vi "Read_fw_info.vi"(8 "error in (no error)":errorcluster, 11 "VISA Refnum in":refnum<visa-resource-name>) -> (0 "error out":errorcluster, 1 "Firmware Version":string, 2 "Hardware":string, 3 "VISA Refnum out":refnum<visa-resource-name>, 5 "Project":string)   [LabVIEW 2019]
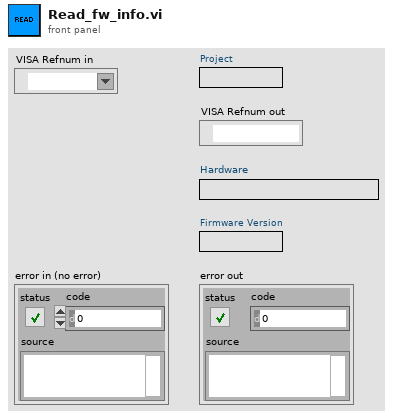
[diagram p1: front panel]
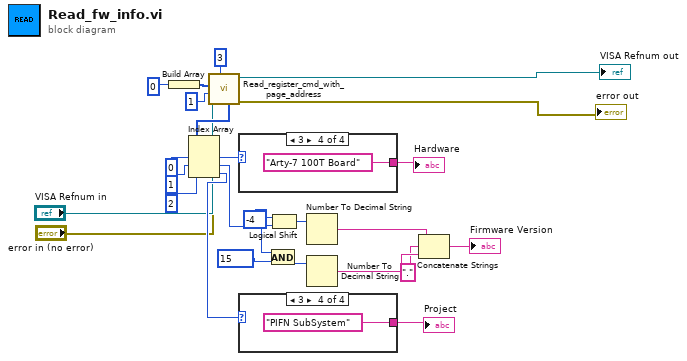
[diagram p0: block diagram]
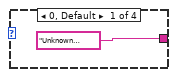
[diagram p2: hidden frame]
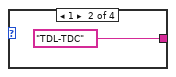
[diagram p3: hidden frame]
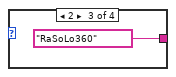
[diagram p4: hidden frame]
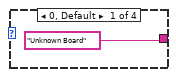
[diagram p5: hidden frame]
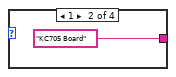
[diagram p6: hidden frame]
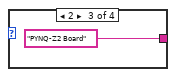
[diagram p7: hidden frame]
diagram:
  n1 = Build Array(u8 0) -> (w1:u8[])
  n2 = call "Read_register_cmd_with_page_address.vi"("Words_to_read"=u16 3, "error in (no error)"="error in (no error)", "Register Address"=u8 1, "Page address"=w1, "VISA Refnum in"="VISA Refnum in") -> ("error out"=→"error out":errorcluster, "VISA Refnum out"=→"VISA Refnum out":refnum<visa-resource-name>, "RdReg Data"=w7:u8[])  [unwired: 4 in]
  n3 = Index Array(array=w7, index #1=0 ("index"), index #2=1 ("index"), index #3=2 ("index")) -> (element #1=w11:u8, element #2=w18:u8, element #3=w22:u8)
  n4 = case shown="3" w11 {
    tunnel: ["Unknown Board" "KC705 Board" "PYNQ-Z2 Board" "Arty-7 100T Board"] -> w12
    frame 0, Default {
    }
    frame 1 {
    }
    frame 2 {
    }
    frame 3 {
    }
  }
  "Hardware" <- w12
  n5 = case shown="3" w22 {
    tunnel: ["Unknown Project" "TDL-TDC" "RaSoLo360" "PIFN SubSystem"] -> w23
    frame 0, Default {
    }
    frame 1 {
    }
    frame 2 {
    }
    frame 3 {
    }
  }
  "Project" <- w23
  n6 = And(x=w18, y=u8 15) -> (x .and. y?=w21:u8)
  n7 = Logical Shift(y=i16 -4, x=w18) -> (x << y=w20:u8)
  n8 = Number To Decimal String(number=w20) -> (decimal integer string=w13:string)  [unwired: 1 in]
  n9 = Number To Decimal String(number=w21) -> (decimal integer string=w15:string)  [unwired: 1 in]
  n10 = Concatenate Strings(w13, "." ("string"), w15) -> (→"Firmware Version":string)
